vi "radom_array-4.21.vi"() -> ()   [LabVIEW 2015]
panel:
  out "最小索引":i32[](array[numeric])
  out "最大索引":i32[](array[numeric])
  out "最小值":dbl
  out "最大值":dbl
  out "Array":dbl[][](array[numeric])
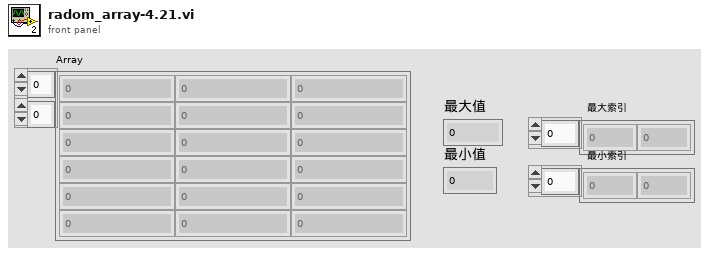
[diagram p1: front panel]
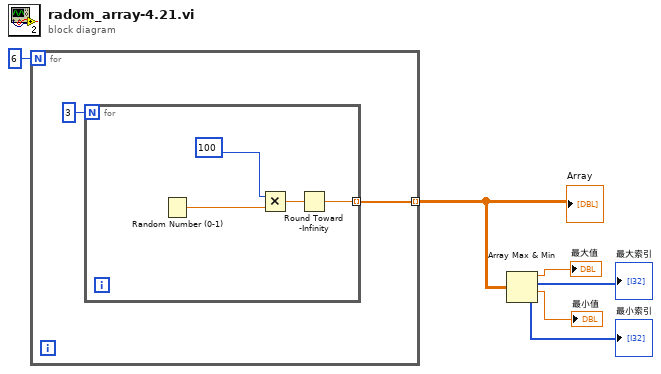
[diagram p0: block diagram]
diagram:
  n1 = for {
    N: 6 -> [_]
    tunnel: [w7] -> w5 mode=indexing
    n2 = for {
      N: 3 -> [_]
      tunnel: [w10] -> w7 mode=indexing
      n3 = Random Number (0-1)() -> (number: 0 to 1=w12:dbl)
      n4 = Multiply(x=100, y=w12) -> (x*y=w9:dbl)
      n5 = Round Toward -Infinity(1:w9) -> (0:w10:dbl)
    }
  }
  "Array" <- w5
  n6 = Array Max & Min(array=w5) -> (max value=→"最大值":dbl, max index (indices)=→"最大索引":i32[], min value=→"最小值":dbl, min index (indices)=→"最小索引":i32[])
